vi "GetScaleData.vi"(8 "error in (no error)":errorcluster, 10 "Grid Descriptor":cluster{"X Step":sgl, "Y Step":sgl, "Unit":T2}={"X Step"=5.0, "Y Step"=5.0, "Unit"=enum."Millimeter"}, 11 "Image Src":T1) -> (0 "error out":errorcluster, 3 "Image":T1(plugin-control))   [LabVIEW 2017]
uses:
  <vilib>/vision/Image Controls.llb/IMAQ Image.ctl
  <vilib>/vision/Calibration.llb/Distortion Model.ctl
  <vilib>/vision/Calibration.llb/Distortion Model Types.ctl
  <vilib>/vision/NI_Vision_Development_Module.lvlib
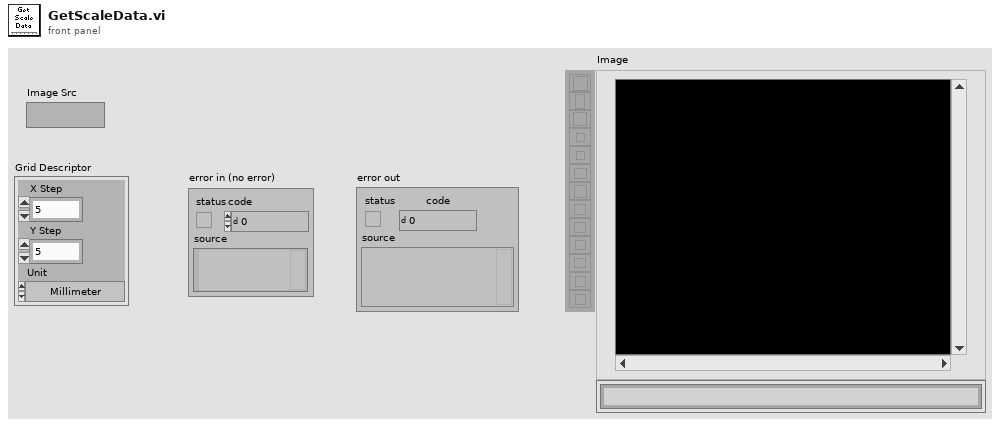
[diagram p1: front panel]
types:
  T1 = typedef "IMAQ Image.ctl" = refnum<image>
  T2 = typedef "Image Unit" = enum32{"Undefined", "Angström", "Micrometer", "Millimeter", "Centimeter", "Meter", "Kilometer", "Microinch", "Inch", "Feet", "Nautical miles", "Standard miles", "Steps"}
  T3 = typedef "Particle Parameters" = i32
  T4 = cluster{"Measurement Parameter":T3, "Range Lower Value":dbl, "Range Upper Value":dbl, "Range":bool, "Measurement Type":bool}[]
  T5 = typedef "Distortion Model.ctl" = cluster{"Distortion Model":T6, "Polynomial Model Setup":cluster{"Radial Coefficient":u32, "Tangential Coefficients ":bool}}
  T6 = typedef "Distortion Model Types.ctl" = i32
  T7 = typedef "Calibration Reference Points.ctl" = cluster{"Pixel Coordinates":cluster{"X":dbl, "Y":dbl}[], "Real World Coordinates":cluster{"X":dbl, "Y":dbl}[], "Unit":T2, "Image Size":cluster{"X":u32, "Y":u32}}
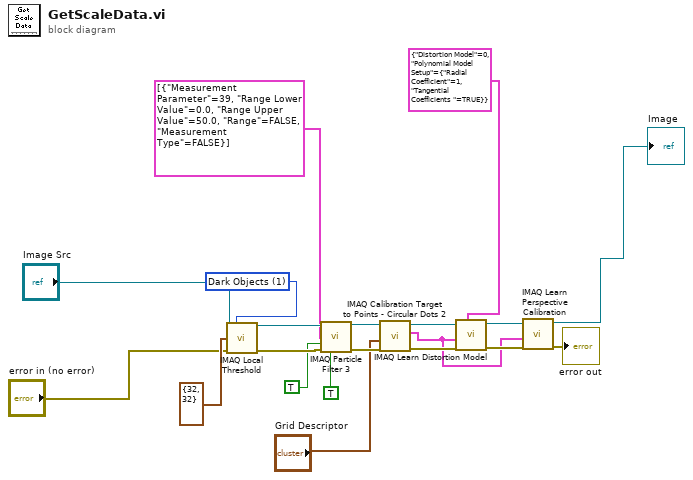
[diagram p0: block diagram]
diagram:
  w20 = u32 1 items=["Bright Objects", "Dark Objects"] ("Look For (Bright Objects)")
  n1 = call "IMAQ Local Threshold"("Image Src"="Image Src", "Look For (Bright Objects)"=w20, "Window Size (32x32)"=cluster{"SizeX":i32, "SizeY":i32} {"SizeX"=32, "SizeY"=32}, "error in (no error)"="error in (no error)") -> ("Image Dst Out"=w14:T1, "error out"=w18:errorcluster)  [unwired: 10 in]
  n2 = call "IMAQ Particle Filter 3"("Image Src"=w14, "Selection Values"=T4 [{"Measurement Parameter"=39, "Range Lower Value"=0.0, "Range Upper Value"=50.0, "Range"=FALSE, "Measurement Type"=FALSE}], "Keep/Remove Particles (F)"=TRUE, "error in (no error)"=w18, "Reject Border? (F)"=TRUE) -> ("Image Dst Out"=w11:T1, "error out"=w17:errorcluster)  [unwired: 8 in, 1 out]
  n3 = call "IMAQ Calibration Target to Points - Circular Dots 2"("error in (no error)"=w17, "Grid Descriptor"="Grid Descriptor", "Target Image"=w11) -> ("error out"=w16:errorcluster, "Reference Points"=w9:T7, "Target Image (dup)"=w10:T1)  [unwired: 6 in]
  n4 = call "IMAQ Learn Distortion Model"("Distortion Model Setup"=T5 {"Distortion Model"=0, "Polynomial Model Setup"={"Radial Coefficient"=1, "Tangential Coefficients "=TRUE}}, "error in (no error)"=w16, "Reference Points"=w9, "Calibration Template Image"=w10) -> ("error out"=w15:errorcluster, "Calibration Template Image Out"=w8:T1)  [unwired: 6 in]
  n5 = call "IMAQ Learn Perspective Calibration"("error in (no error)"=w15, "Reference Points"=w9, "Calibration Template Image"=w8) -> ("error out"=→"error out":errorcluster, "Calibration Template Image Out"=→"Image":T1)  [unwired: 7 in]
